vi "Close.vi"(8 "error in":errorcluster, 11 "Sourcegrid in":refnum<class "SourceGrid.lvclass">) -> (0 "error out":errorcluster, 3 "Sourcegrid out":refnum<class "SourceGrid.lvclass">)   [LabVIEW 2024, in "SourceGrid.lvlib" / "SourceGrid.lvclass"]
uses:
  SourceGrid.lvclass
  SourceGrid.lvclass/SourceGrid.ctl
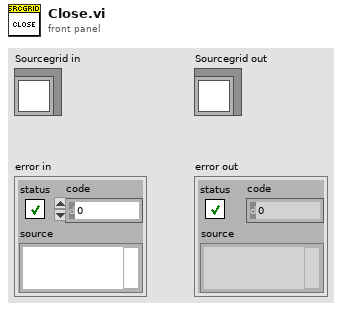
[diagram p1: front panel]
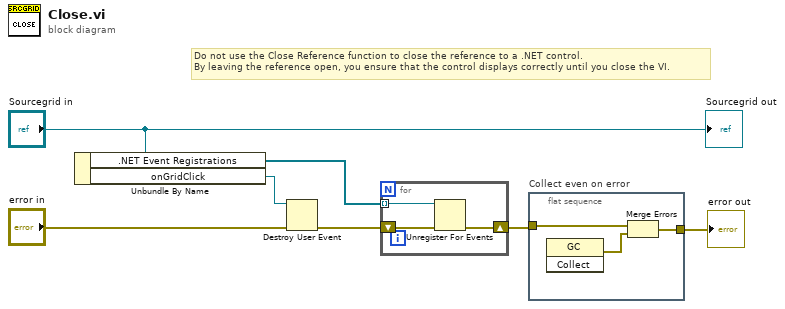
[diagram p0: block diagram]
diagram:
  # "Do not use the Close Reference function to close the reference to a .NET control.\nBy leaving the reference open, you ensure that the control displays correctly until you close the VI."
  n1 = Unbundle By Name("Sourcegrid in") -> (".NET Event Registrations"=w6:refnum<k27>[], "onGridClick"=w3:refnum<user-event>)
  n2 = Destroy User Event(user event=w3, error in="error in") -> (error out=w2:errorcluster)
  n3 = for {
    shift-right: [w9] -> w5
    shift-left: w2 -> [w10]
    tunnel: w6 -> [w8] mode=indexing
    n4 = Unregister For Events(event registration refnum=w8, error in=w10) -> (error out=w9:errorcluster)
  }
  n5 = flat-sequence "Collect even on error" {
    tunnel: [w12] -> w4
    tunnel: w5 -> [w11]
    frame #0 {
      n6 = invoke class="GC" method="Collect"() -> (error out=w13:errorcluster)  [unwired: 3 in, 2 out]
      n7 = Merge Errors(w11, w13) -> (w12:errorcluster)
    }
  }
  "error out" <- w4
  "Sourcegrid out" <- "Sourcegrid in"
